vi "Setup default bools.vi"(7 "appended array":refnum<vi>[](array[refnum]), 8 "error in (no error)":errorcluster, 9 "Property Values":bool[](array[boolean]), 10 "Property Names":string[](array[string]), 11 "Item Ref In":T1 format="%.0x") -> (0 "error out":errorcluster, 3 "Item Ref out":T1 format="%.0x")   [LabVIEW 2023, in "Embedded TDMS Logger System Explorer.lvlib"]
uses:
  <vilib>/NI VeriStand/Custom Device API/Custom Device Item Ref.ctl
  Embedded TDMS Logger System Explorer.lvlib
  <vilib>/NI VeriStand/Custom Device API/Custom Device API.lvlib
  <vilib>/NI VeriStand/Custom Device API/Get Item Property (Boolean).vi
  <vilib>/NI VeriStand/Custom Device API/Set Item Property (Boolean).vi
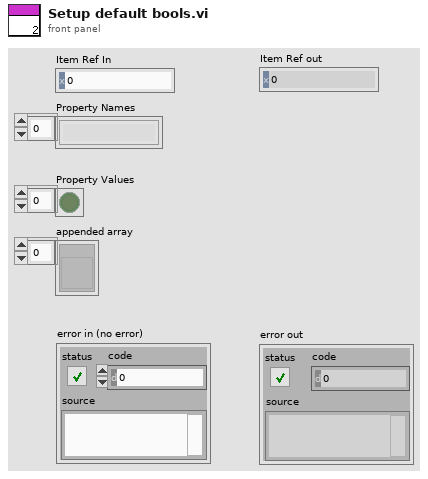
[diagram p1: front panel]
types:
  T1 = typedef "Custom Device API.lvlib/Custom Device Item Ref.ctl" = u64
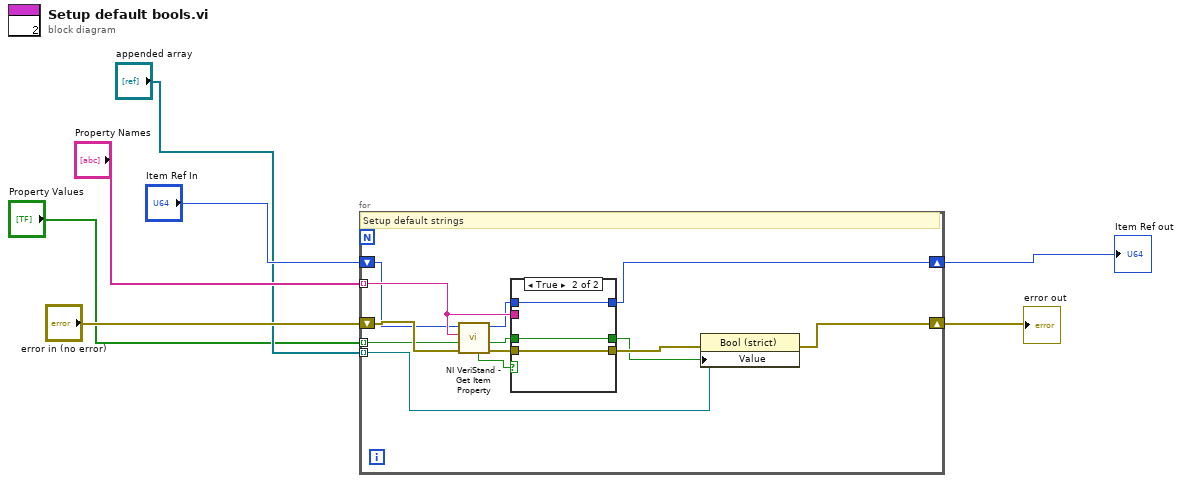
[diagram p0: block diagram]
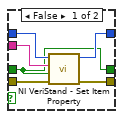
[diagram p2: hidden frame]
diagram:
  n1 = for {
    tunnel: "Property Names" -> [w15] mode=indexing
    shift-right: [w17] -> w4
    shift-left: "error in (no error)" -> [w13]
    shift-right: [w20] -> w6
    shift-left: "Item Ref In" -> [w12]
    tunnel: "appended array" -> [w19] mode=indexing
    tunnel: "Property Values" -> [w8] mode=indexing
    # "Setup default strings"
    n2 = call-poly <vilib>:"NI VeriStand - Get Item Property.vi"("error in (no error)"=w13, "Default Value"=w8, "Property Name"=w15, "Item Ref in"=w12) -> ("error out"=w14:errorcluster, "Value"=w10:bool, "Item Ref out"=w11:T1, "Found?"=w16:bool)  [unwired: 4 in]
    n3 = case shown="True" w16 {
      tunnel: [w26 w29] -> w20
      tunnel: w11 -> [w25 w29]
      tunnel: [w24 w28] -> w18
      tunnel: w15 -> [w23 _]
      tunnel: w14 -> [w22 w28]
      tunnel: w10 -> [w21 w27]
      tunnel: [w21 w27] -> w9
      frame False {
        n4 = call-poly <vilib>:"NI VeriStand - Set Item Property.vi"("error in (no error)"=w22, "Value"=w21, "Property Name"=w23, "Item Ref in"=w25) -> ("error out"=w24:errorcluster, "Item Ref out"=w26:T1)  [unwired: 5 in, 1 out]
      }
      frame True {
      }
    }
    n5 = property class="Bool (strict)"(reference=w19, error in=w18, "Value"=w9) -> (error out=w17:errorcluster)  [unwired: 1 out]
  }
  "Item Ref out" <- w6
  "error out" <- w4
